vi "Button Handler.vi"(8 "error in (no error)":errorcluster, 11 "Buttons":bool[](array[boolean])) -> (0 "error out":errorcluster)   [LabVIEW 2014]
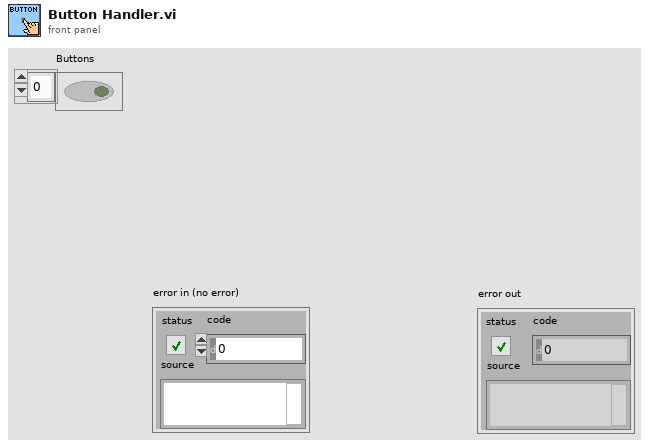
[diagram p1: front panel]
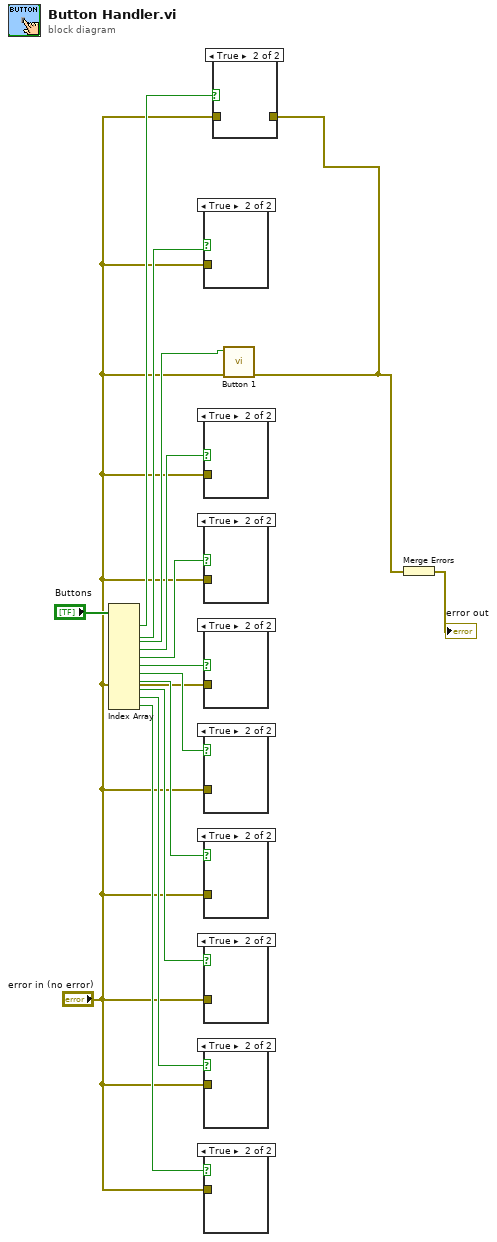
[diagram p0: block diagram]
diagram:
  n1 = Index Array(array="Buttons") -> (element #1=w3:bool, element #2=w14:bool, element #3=w2:bool, element #4=w13:bool, element #5=w12:bool, element #6=w11:bool, element #7=w10:bool, element #8=w9:bool, element #9=w8:bool, element #10=w7:bool, element #11=w6:bool)  [unwired: 11 in]
  n2 = case shown="True" w14 {
    tunnel: "error in (no error)" -> [_ _]
    frame False {
    }
    frame True {
    }
  }
  n3 = case shown="True" w13 {
    tunnel: "error in (no error)" -> [_ _]
    frame False {
    }
    frame True {
    }
  }
  n4 = case shown="True" w12 {
    tunnel: "error in (no error)" -> [_ _]
    frame False {
    }
    frame True {
    }
  }
  n5 = case shown="True" w11 {
    tunnel: "error in (no error)" -> [_ _]
    frame False {
    }
    frame True {
    }
  }
  n6 = case shown="True" w10 {
    tunnel: "error in (no error)" -> [_ _]
    frame False {
    }
    frame True {
    }
  }
  n7 = case shown="True" w9 {
    tunnel: "error in (no error)" -> [_ _]
    frame False {
    }
    frame True {
    }
  }
  n8 = case shown="True" w8 {
    tunnel: "error in (no error)" -> [_ _]
    frame False {
    }
    frame True {
    }
  }
  n9 = case shown="True" w7 {
    tunnel: "error in (no error)" -> [_ _]
    frame False {
    }
    frame True {
    }
  }
  n10 = case shown="True" w6 {
    tunnel: "error in (no error)" -> [_ _]
    frame False {
    }
    frame True {
    }
  }
  n11 = call "Button 1.vi"("error in (no error)"="error in (no error)", "button value"=w2) -> ("error out"=w4:errorcluster)  [unwired: 9 in]
  n12 = case shown="True" w3 {
    tunnel: "error in (no error)" -> [_ _]
    tunnel: w4 -> [_ _]
    frame False {
    }
    frame True {
    }
  }
  n13 = Merge Errors(w4) -> (→"error out":errorcluster)
